vi "getCallerVIpath.vi"() -> (1 "calling VI's  parent path":path, 2 "calling VI's absolute path":path)   [LabVIEW 2017]
doc: "SciScan 1.2 160622"
panel:
  out "error out":errorcluster
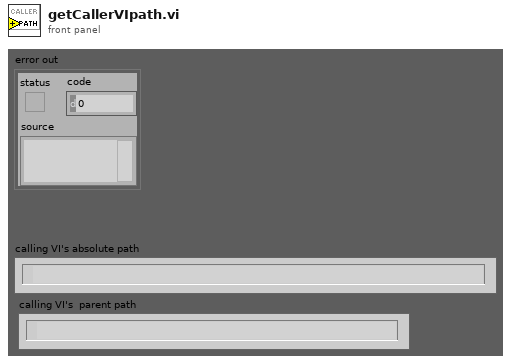
[diagram p1: front panel]
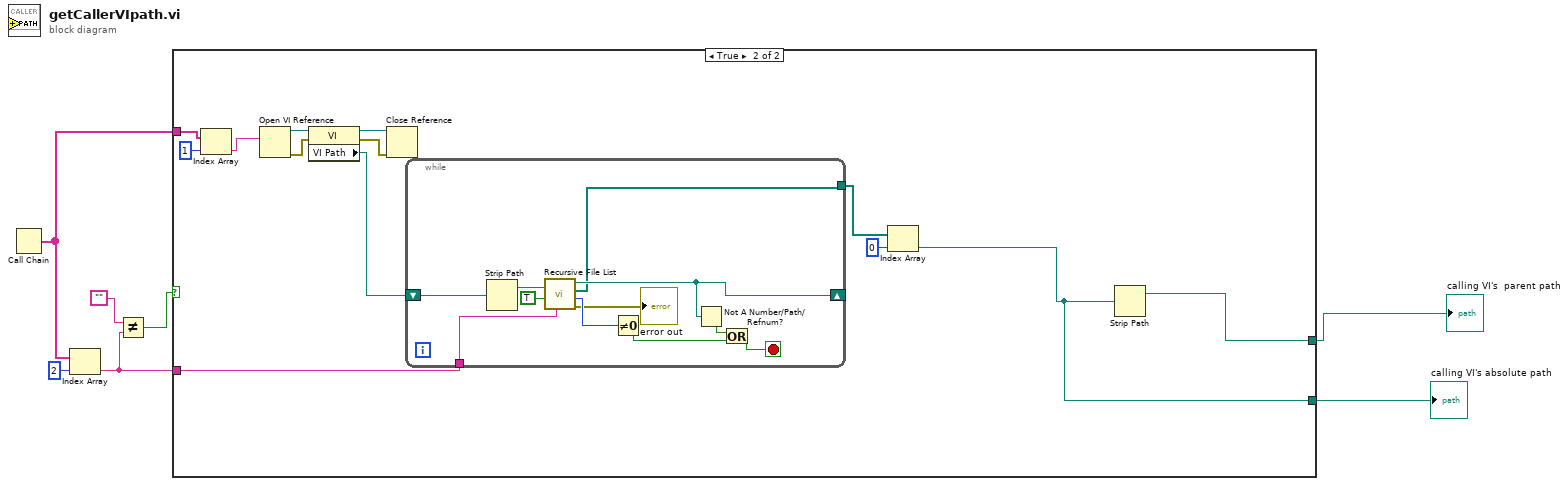
[diagram p0: block diagram]
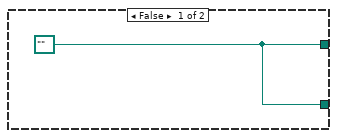
[diagram p2: hidden frame]
diagram:
  n1 = Call Chain() -> (call chain=w7:string[])
  n2 = Index Array(array=w7, index=2) -> (element=w4:string)
  n3 = Not Equal?(x="", y=w4) -> (x != y?=w3:bool)
  n4 = case shown="True" w3 {
    tunnel: w7 -> [_ w14]
    tunnel: w4 -> [_ w13]
    tunnel: [w8 w12] -> w6
    tunnel: [w8 w9] -> w1
    frame False {
      w8 = path "" ("stripped path")
    }
    frame True {
      n5 = Index Array(array=w14, index=1) -> (element=w15:string)
      n6 = Open VI Reference(vi path=w15) -> (vi reference=w21:refnum<vi>, error out=w20:errorcluster)  [unwired: 5 in]
      n7 = property class="VI"(reference=w21, error in=w20) -> (reference out=w19:refnum<vi>, error out=w18:errorcluster, "VI Path"=w17:path)
      n8 = Close Reference(reference=w19, error in (no error)=w18) -> ()  [unwired: 1 out]
      n9 = while {
        tunnel: w13 -> [w23]
        shift-right: [w27] -> _
        shift-left: w17 -> [w32]
        tunnel: [w22] -> w11
        stop <- w26 stop-if-true
        n10 = Strip Path(path=w32) -> (stripped path=w31:path)  [unwired: 1 out]
        n11 = call <vilib>:"Recursive File List.vi"("pattern"=w23, "Continue Recursing on Error? (F)"=TRUE, "Folder Path"=w31) -> ("error out"=→"error out":errorcluster, "Number of Files"=w30:i32, "All Files in Dir"=w22:path[], "dup Folder Path"=w27:path)  [unwired: 4 in, 1 out]
        n12 = Not Equal To 0?(x=w30) -> (x != 0?=w29:bool)
        n13 = Not A Number/Path/Refnum?(number/path/refnum=w27) -> (NaN/Path/Refnum?=w25:bool)
        n14 = Or(x=w25, y=w29) -> (x .or. y?=w26:bool)
      }
      n15 = Index Array(array=w11, index=0) -> (element=w9:path)
      n16 = Strip Path(path=w9) -> (stripped path=w12:path)  [unwired: 1 out]
    }
  }
  "calling VI's  parent path" <- w6
  "calling VI's absolute path" <- w1
